vi "B_sweep_3ch_DR_v2.1.vi"(1 "name or relative path":string="Bsweeps_lockin_500mK_Vbg2.0V", 3 "description":string="SA02657K.20130302\ntemp=500mK\nVbg=1.9V\n25Oe/s scan rate", 5 "Stop":bool, 8 "slow scan through zero?":bool, 11 "sec to stablize B":u32=10, 15 "B Start (Oe)":dbl=-10000.0, 16 "B End (Oe)":dbl=10000.0, 17 "B Scan (Oe/sec)":dbl=25.0) -> (0 "Pickering":string="I-:5\nV2+:28\nI+:2\nV1+:3\nV-:4\nV2-:4\n", 10 "Zx 2":cluster{"Y":dbl[], "Y":dbl[]}(graph), 12 "Zx":cluster{"Y":dbl[], "Y":dbl[]}(graph), 13 "T":cluster{"Y":dbl[], "Y":dbl[]}(graph), 18 "Y Channel":cluster{"Y":dbl[], "Y":dbl[]}(graph), 19 "X Channel":cluster{"Y":dbl[], "Y":dbl[]}(graph))   [LabVIEW 2011]
uses:
  SubVI/ITX_Global.vi
  DAQ-lockin-SubVI/Source/Lock-in Globles.vi
panel:
  out "Current field (Oe)":dbl=9993.39
  in  "Tab Control":T1(tab)
  in  "Lock-in #":u16(ring) items=["Lock-in #1", "Lock-in #2", "Lock-in #3", "Lock-in #4"]
  in  "Lock-in # 3":u16(ring)=2 items=["Lock-in #1", "Lock-in #2", "Lock-in #3", "Lock-in #4"]
  in  "Lock-in # 4":u16(ring)=3 items=["Lock-in #1", "Lock-in #2", "Lock-in #3", "Lock-in #4"]
  in  "Device image":path=path "C:/Experiments/2011-summer Superconductivity-Spin Hall/Device images/SA02657K_20130302.png"
  out "Last Scan Image":T2(plugin-control)
  in  "Initial Rate (Oe/s)":i32=25
  in  "Stop Lockin":bool
  out "X 3":cluster{"Y":dbl[], "Y":dbl[]}(graph)
  out "Y 3":cluster{"Y":dbl[], "Y":dbl[]}(graph)
  out "X 4":cluster{"Y":dbl[], "Y":dbl[]}(graph)
  out "Y4":cluster{"Y":dbl[], "Y":dbl[]}(graph)
  out "Zy":cluster{"Y":dbl[], "Y":dbl[]}(graph)
  out "Zy 2":cluster{"Y":dbl[], "Y":dbl[]}(graph)
  # "yes"
  # "no"
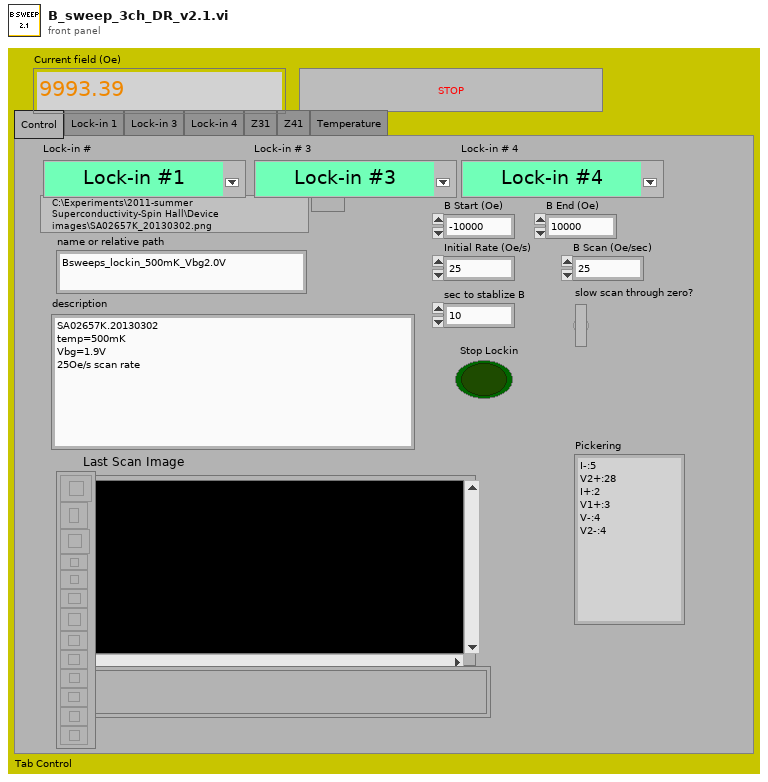
[diagram p1: front panel]
types:
  T1 = enum32{"Control", "Lock-in 1", "Lock-in 3", "Lock-in 4", "Z31", "Z41", "Temperature"}
  T2 = typedef "IMAQ Image.ctl" = refnum<image>
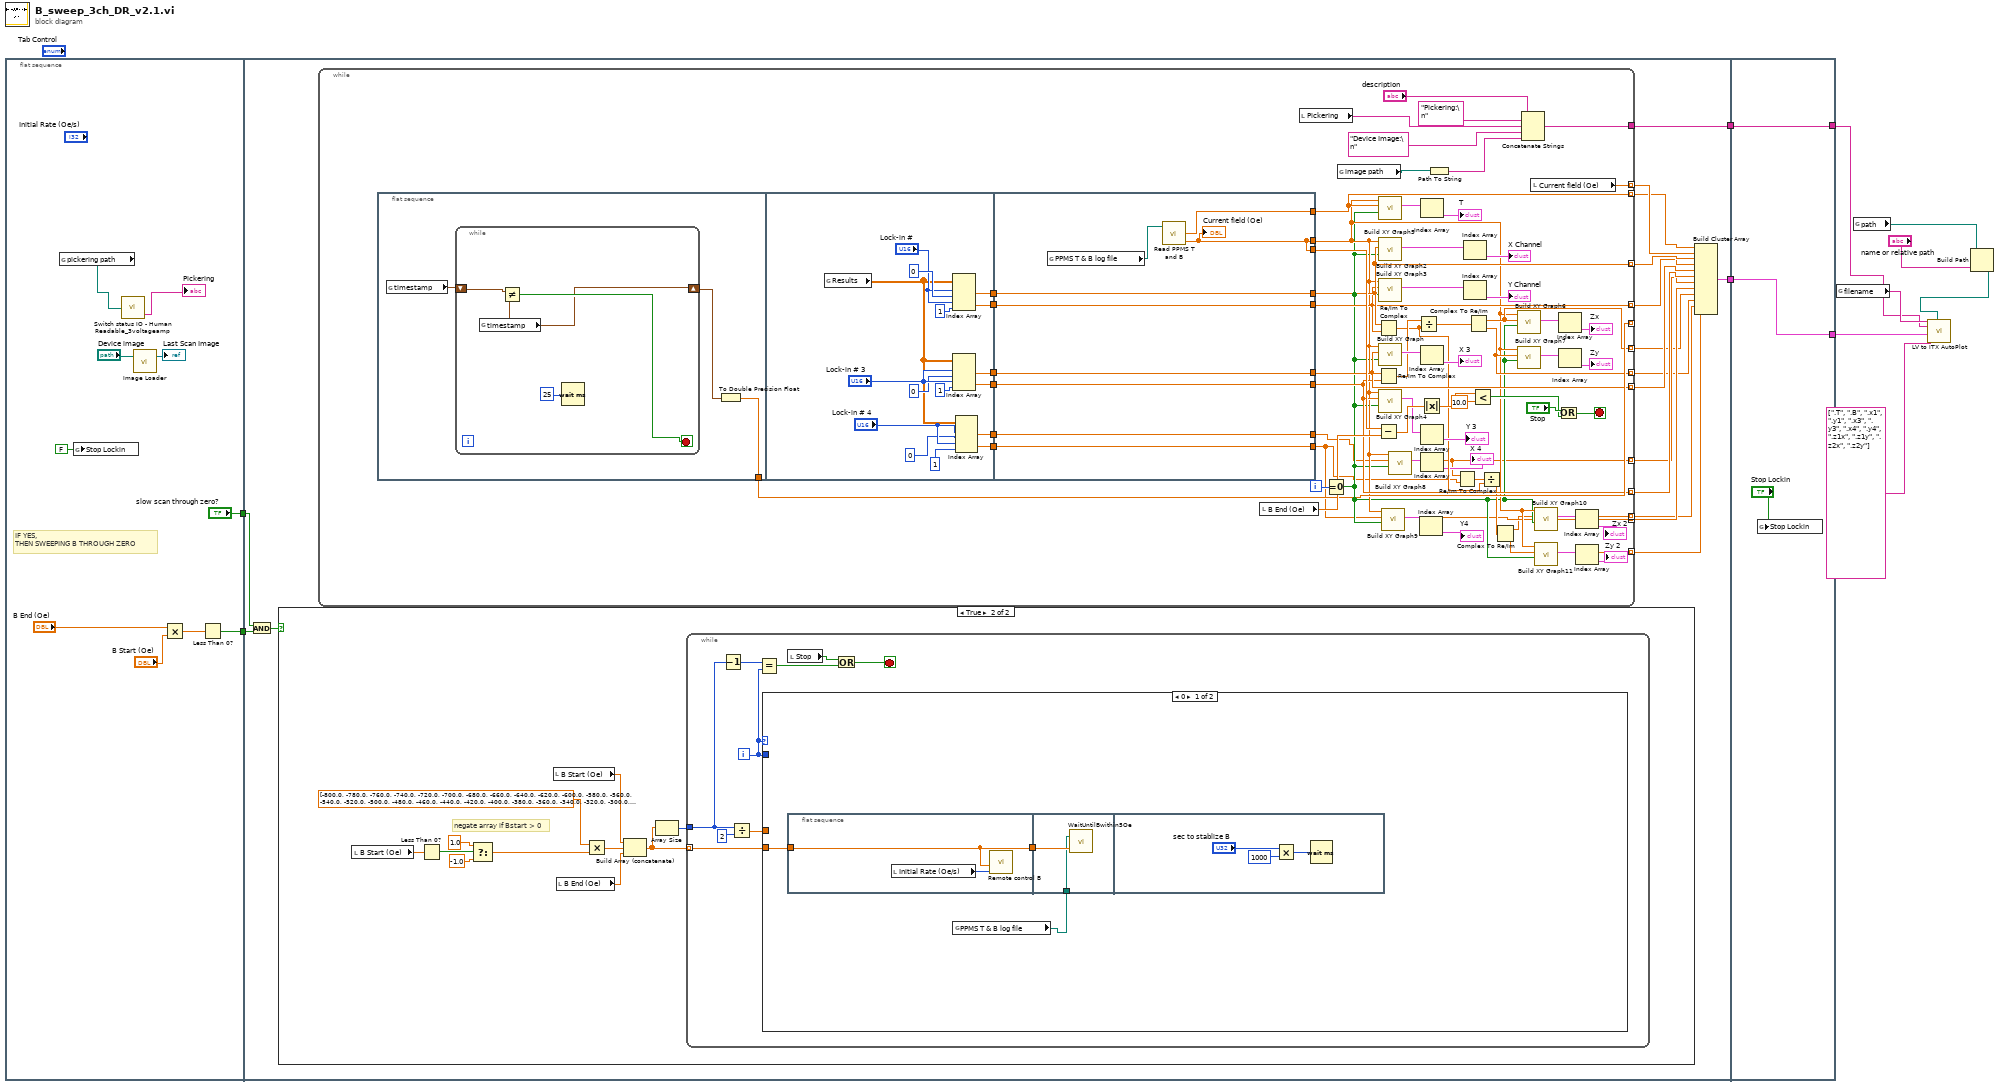
[diagram p0: block diagram]
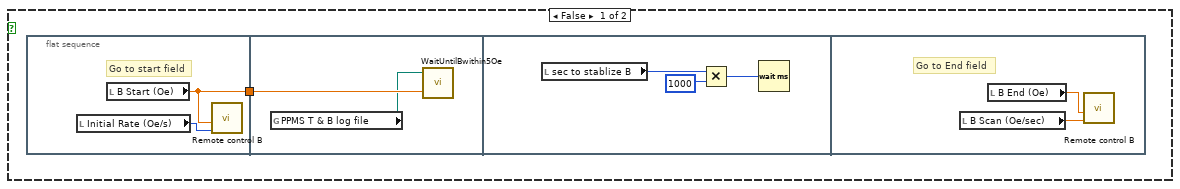
[diagram p2: hidden frame]
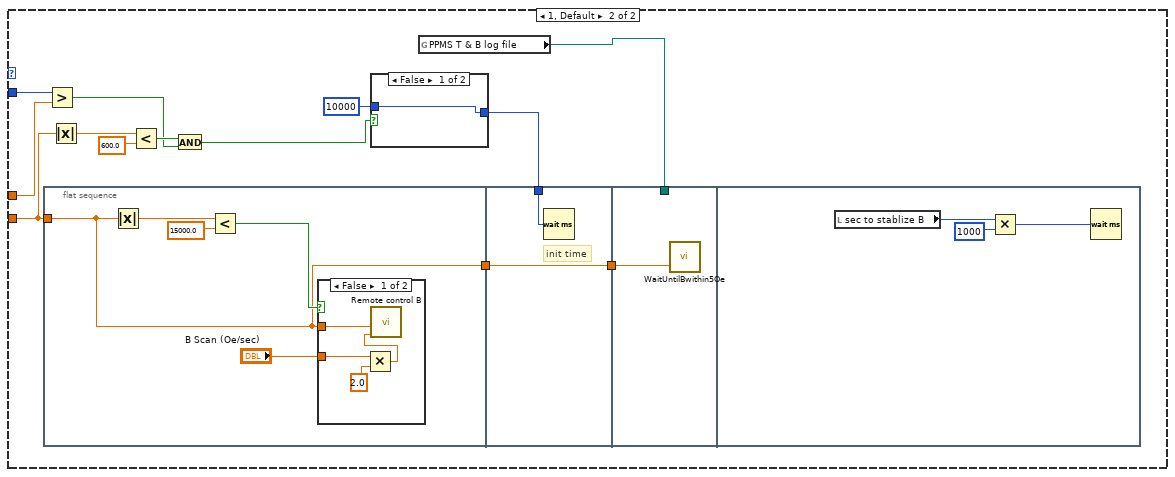
[diagram p3: hidden frame]
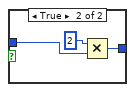
[diagram p4: hidden frame]
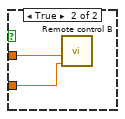
[diagram p5: hidden frame]
diagram:
  n1 = flat-sequence {
    tunnel: [w20] -> w11
    tunnel: ["slow scan through zero?"] -> w10
    tunnel: w11 -> [w38]
    tunnel: w10 -> [w37]
    tunnel: [w35] -> w7
    tunnel: [w22] -> w2
    tunnel: [w211] -> w4
    tunnel: w7 -> [w211]
    tunnel: [w209] -> w3
    tunnel: w2 -> [w209]
    frame #0 {
      # "IF YES,\nTHEN SWEEPING B THROUGH ZERO"
      n2 = global read "ITX_Global.vi" "pickering path"() -> (w13:path)
      n3 = global write "Lock-in Globles.vi" "Stop Lockin"(FALSE ("Stop Lockin")) -> ()
      n4 = call <userlib>:"Switch status IO - Human Readable_3voltageamp.vi"("Switch status"=w13) -> ("String"=→"Pickering":string)  [unwired: 3 in]
      n5 = call "Image Loader.vi"("File Path"="Device image") -> ("Last Scan Image"=→"Last Scan Image":T2)  [unwired: 2 in]
      n6 = Multiply(x="B End (Oe)", y="B Start (Oe)") -> (x*y=w21:dbl)
      n7 = Less Than 0?(x=w21) -> (x < 0?=w20:bool)
    }
    frame #1 {
      n8 = And(x=w37, y=w38) -> (x .and. y?=w36:bool)
      n9 = case shown="True" w36 {
        frame False {
          n10 = flat-sequence {
            tunnel: [w40] -> w39
            tunnel: w39 -> [w43]
            frame #0 {
              # "Go to start field"
              n11 = local read "Initial Rate (Oe/s)"() -> (w41:i32)
              n12 = local read "B Start (Oe)"() -> (w40:dbl)
              n13 = call "Remote control B.vi"("Rate (Oe/s)"=w41, "Field (Oe)"=w40) -> ()  [unwired: 7 in, 1 out]
            }
            frame #1 {
              n14 = global read "ITX_Global.vi" "PPMS T & B log file"() -> (w42:path)
              n15 = call "WaitUntilBwithin5Oe.vi"("Target Field (Oe)"=w43, "PPMS T & B log file"=w42) -> ()  [unwired: 2 in]
            }
            frame #2 {
              n16 = local read "sec to stablize B"() -> (w44:u32)
              n17 = Multiply(x=w44, y=u32 1000) -> (x*y=w45:u32)
              n18 = Wait (ms)(milliseconds to wait=w45) -> ()  [unwired: 1 out]
            }
            frame #3 {
              # "Go to End field"
              n19 = local read "B Scan (Oe/sec)"() -> (w47:dbl)
              n20 = local read "B End (Oe)"() -> (w48:dbl)
              n21 = call "Remote control B.vi"("Rate (Oe/s)"=w47, "Field (Oe)"=w48) -> ()  [unwired: 7 in, 1 out]
            }
          }
        }
        frame True {
          # "negate array if Bstart > 0"
          n22 = local read "B Start (Oe)"() -> (w59:dbl)
          n23 = Less Than 0?(x=w59) -> (x < 0?=w57:bool)
          n24 = Select(t=1.0, s=w57, f=-1.0) -> (s? t:f=w56:dbl)
          n25 = local read "B Start (Oe)"() -> (w51:dbl)
          n26 = local read "B End (Oe)"() -> (w52:dbl)
          n27 = Multiply(x=dbl[] [-800.0, -780.0, -760.0, -740.0, -720.0, -700.0, -680.0, -660.0, -640.0, -620.0, -600.0, -580.0, -560.0, -540.0, -520.0, -500.0, -480.0, -460.0, -440.0, -420.0, -400.0, -380.0, -360.0, -340.0, -320.0, -300.0, -280.0, -260.0, -240.0, -220.0, -200.0, -190.0, -180.0, -170.0, -160.0, -150.0, -140.0, -130.0, -120.0, -110.0, -100.0, -90.0, -80.0, -70.0, -60.0, -50.0, -40.0, -30.0, -20.0, -10.0, 0.0, 10.0, 20.0, 30.0, 40.0, 50.0, 60.0, 70.0, 80.0, 90.0, 100.0, 110.0, 120.0, 130.0, 140.0, 150.0, 160.0, 170.0, 180.0, 190.0, 200.0, 220.0, 240.0, 260.0, 280.0, 300.0, 320.0, 340.0, 360.0, 380.0, 400.0, 420.0, 440.0, 460.0, 480.0, 500.0, 520.0, 540.0, 560.0, 580.0, 600.0, 620.0, 640.0, 660.0, 680.0, 700.0, 720.0, 740.0, 760.0, 780.0, 800.0], y=w56) -> (x*y=w53:dbl[])
          n28 = Build Array (concatenate)(w51, w53, w52) -> (w50:dbl[])
          n29 = Array Size(array=w50) -> (size(s)=w49:i32)
          n30 = while {
            tunnel: w50 -> [w68] mode=indexing
            tunnel: w49 -> [w63]
            i -> [w60]
            stop <- w64 stop-if-true
            n31 = Decrement(x=w63) -> (x-1=w67:i32)
            n32 = Divide(x=w63, y=2) -> (x/y=w61:dbl)
            n33 = Equal?(x=w67, y=w60) -> (x = y?=w66:bool)
            n34 = case shown="0" w60 {
              tunnel: w68 -> [w70 w89]
              tunnel: w61 -> [_ w85]
              tunnel: w60 -> [_ w84]
              frame 0 {
                n35 = flat-sequence {
                  tunnel: w70 -> [w73]
                  tunnel: [w73] -> w71
                  tunnel: w69 -> [w74]
                  tunnel: w71 -> [w75]
                  frame #0 {
                    n36 = local read "Initial Rate (Oe/s)"() -> (w72:i32)
                    n37 = call "Remote control B.vi"("Rate (Oe/s)"=w72, "Field (Oe)"=w73) -> ()  [unwired: 7 in, 1 out]
                  }
                  frame #1 {
                    n38 = call "WaitUntilBwithin5Oe.vi"("Target Field (Oe)"=w75, "PPMS T & B log file"=w74) -> ()  [unwired: 2 in]
                  }
                  frame #2 {
                    n39 = Multiply(x="sec to stablize B", y=u32 1000) -> (x*y=w77:u32)
                    n40 = Wait (ms)(milliseconds to wait=w77) -> ()  [unwired: 1 out]
                  }
                }
                n41 = global read "ITX_Global.vi" "PPMS T & B log file"() -> (w69:path)
              }
              frame 1, Default {
                n42 = flat-sequence {
                  tunnel: w89 -> [w97]
                  tunnel: [w97] -> w91
                  tunnel: w91 -> [w108]
                  tunnel: [w108] -> w90
                  tunnel: w80 -> [w107]
                  tunnel: w79 -> [_]
                  tunnel: w90 -> [w109]
                  frame #0 {
                    n43 = Absolute Value(x=w97) -> (abs(x)=w96:dbl)
                    n44 = Less?(x=w96, y=15000.0) -> (x < y?=w98:bool)
                    n45 = case shown="False" w98 {
                      tunnel: w97 -> [w104 w106]
                      tunnel: "B Scan (Oe/sec)" -> [w103 w105]
                      frame False {
                        n46 = Multiply(x=w103, y=2.0) -> (x*y=w101:dbl)
                        n47 = call "Remote control B.vi"("Rate (Oe/s)"=w101, "Field (Oe)"=w104) -> ()  [unwired: 7 in, 1 out]
                      }
                      frame True {
                        n48 = call "Remote control B.vi"("Rate (Oe/s)"=w105, "Field (Oe)"=w106) -> ()  [unwired: 7 in, 1 out]
                      }
                    }
                  }
                  frame #1 {
                    # "init time"
                    n49 = Wait (ms)(milliseconds to wait=w107) -> ()  [unwired: 1 out]
                  }
                  frame #2 {
                    n50 = call "WaitUntilBwithin5Oe.vi"("Target Field (Oe)"=w109) -> ()  [unwired: 3 in]
                  }
                  frame #3 {
                    n51 = local read "sec to stablize B"() -> (w110:u32)
                    n52 = Multiply(x=w110, y=u32 1000) -> (x*y=w111:u32)
                    n53 = Wait (ms)(milliseconds to wait=w111) -> ()  [unwired: 1 out]
                  }
                }
                n54 = Greater?(x=w84, y=w85) -> (0:w83:bool)
                n55 = Absolute Value(x=w89) -> (abs(x)=w86:dbl)
                n56 = Less?(x=w86, y=600.0) -> (x < y?=w87:bool)
                n57 = And(x=w87, y=w83) -> (x .and. y?=w82:bool)
                n58 = case shown="False" w82 {
                  tunnel: u32 10000 ("y") -> [w92 w95]
                  tunnel: [w92 w93] -> w80
                  frame False {
                  }
                  frame True {
                    n59 = Multiply(x=u32 2, y=w95) -> (x*y=w93:u32)
                  }
                }
                n60 = global read "ITX_Global.vi" "PPMS T & B log file"() -> (w79:path)
              }
            }
            n61 = local read "Stop"() -> (w65:bool)
            n62 = Or(x=w65, y=w66) -> (x .or. y?=w64:bool)
          }
        }
      }
      n63 = while {
        tunnel: [w147] -> _ mode=indexing
        tunnel: [w146] -> w33 mode=indexing
        tunnel: [w145] -> w34 mode=indexing
        tunnel: [w144] -> w32 mode=indexing
        tunnel: [w143] -> w30 mode=indexing
        tunnel: [w142] -> w31 mode=indexing
        tunnel: [w141] -> w29 mode=indexing
        tunnel: [w140] -> w26 mode=indexing
        tunnel: [w139] -> w25 mode=indexing
        tunnel: [w117] -> w35
        tunnel: [w116] -> w28 mode=indexing
        tunnel: [w115] -> w27 mode=indexing
        tunnel: [w114] -> w24 mode=indexing
        tunnel: [w113] -> w23 mode=indexing
        i -> [w176]
        stop <- w169 stop-if-true
        n64 = flat-sequence {
          tunnel: [w179] -> w147
          tunnel: [w196] -> w151
          tunnel: [w195] -> w150
          tunnel: [w191] -> w149
          tunnel: [w190] -> w148
          tunnel: [w185] -> w138
          tunnel: [w184] -> w137
          tunnel: [w203] -> w127
          tunnel: [w203] -> w159
          tunnel: w151 -> [w208]
          tunnel: [w208] -> w142
          tunnel: w150 -> [w207]
          tunnel: [w207] -> w144
          tunnel: [w206] -> w143
          tunnel: w149 -> [w206]
          tunnel: w148 -> [w205]
          tunnel: [w205] -> w141
          tunnel: [w204] -> w146
          tunnel: [w202] -> w116
          tunnel: w138 -> [w202]
          tunnel: [w201] -> w115
          tunnel: w137 -> [w201]
          frame #0 {
            n65 = global read "Lock-in Globles.vi" "timestamp"() -> (w178:timestamp)
            n66 = while {
              shift-right: [w181] -> w177
              shift-left: w178 -> [w183]
              stop <- w182 stop-if-true
              n67 = global read "Lock-in Globles.vi" "timestamp"() -> (w181:timestamp)
              n68 = Not Equal?(x=w183, y=w181) -> (x != y?=w182:bool)
              n69 = Wait (ms)(milliseconds to wait=u32 25) -> ()  [unwired: 1 out]
            }
            n70 = To Double Precision Float(number=w177) -> (double precision float=w179:dbl)
          }
          frame #1 {
            n71 = global read "Lock-in Globles.vi" "Results"() -> (w186:dbl[][])
            n72 = Index Array(array=w186, index (row) #1="Lock-in #", index (col) #1=0 ("disabled index (col)"), index (row) #2="Lock-in #", index (col) #2=1 ("disabled index (col)")) -> (element #1=w195:dbl, element #2=w196:dbl)
            n73 = Index Array(array=w186, index (row) #1="Lock-in # 3", index (col) #1=0 ("disabled index (col)"), index (row) #2="Lock-in # 3", index (col) #2=1 ("disabled index (col)")) -> (element #1=w191:dbl, element #2=w190:dbl)
            n74 = Index Array(array=w186, index (row) #1="Lock-in # 4", index (col) #1=0 ("disabled index (col)"), index (row) #2="Lock-in # 4", index (col) #2=1 ("disabled index (col)")) -> (element #1=w185:dbl, element #2=w184:dbl)
          }
          frame #2 {
            n75 = global read "ITX_Global.vi" "PPMS T & B log file"() -> (w200:path)
            n76 = call "Read PPMS T and B.vi"("file (use dialog)"=w200) -> ("Field"=w203:dbl, "Temperature"=w204:dbl)  [unwired: 2 in, 1 out]
            "Current field (Oe)" <- w203
          }
        }
        n77 = local read "B End (Oe)"() -> (w160:dbl)
        n78 = local read "Pickering"() -> (w119:string)
        n79 = Equal To 0?(x=w176) -> (x = 0?=w126:bool)
        n80 = global read "ITX_Global.vi" "image path"() -> (w118:path)
        n81 = Re/Im To Complex(1:w142, 2:w144) -> (0:w135:cdb)
        n82 = Re/Im To Complex(1:w141, 2:w143) -> (0:w164:cdb)
        n83 = Subtract(x=w159, y=w160) -> (x-y=w174:dbl)
        n84 = call "Build XY Graph5"("Reset"=w126, "Y Input"=w146, "X Input"=w127) -> ("XY Graph"=w165:cluster{"Y":dbl[], "Y":dbl[]}[])  [unwired: 2 in, 6 out]
        n85 = call "Build XY Graph2"("Reset"=w126, "Y Input"=w144, "X Input"=w127) -> ("XY Graph"=w170:cluster{"Y":dbl[], "Y":dbl[]}[])  [unwired: 2 in, 6 out]
        n86 = call "Build XY Graph3"("Reset"=w126, "Y Input"=w142, "X Input"=w127) -> ("XY Graph"=w171:cluster{"Y":dbl[], "Y":dbl[]}[])  [unwired: 2 in, 6 out]
        n87 = call "Build XY Graph"("Reset"=w126, "Y Input"=w143, "X Input"=w127) -> ("XY Graph"=w167:cluster{"Y":dbl[], "Y":dbl[]}[])  [unwired: 2 in, 6 out]
        n88 = call "Build XY Graph4"("Reset"=w126, "Y Input"=w141, "X Input"=w127) -> ("XY Graph"=w166:cluster{"Y":dbl[], "Y":dbl[]}[])  [unwired: 2 in, 6 out]
        n89 = call "Build XY Graph9"("Reset"=w126, "Y Input"=w115, "X Input"=w127) -> ("XY Graph"=w131:cluster{"Y":dbl[], "Y":dbl[]}[])  [unwired: 2 in, 6 out]
        n90 = call "Build XY Graph8"("Reset"=w126, "Y Input"=w116, "X Input"=w127) -> ("XY Graph"=w133:cluster{"Y":dbl[], "Y":dbl[]}[])  [unwired: 2 in, 6 out]
        n91 = Divide(x=w164, y=w135) -> (x/y=w163:cdb)
        n92 = Index Array(array=w131) -> (element=→"Y4":cluster{"Y":dbl[], "Y":dbl[]})  [unwired: 1 in]
        n93 = Index Array(array=w165) -> (element=→"T":cluster{"Y":dbl[], "Y":dbl[]})  [unwired: 1 in]
        n94 = Index Array(array=w167) -> (element=→"X 3":cluster{"Y":dbl[], "Y":dbl[]})  [unwired: 1 in]
        n95 = Absolute Value(x=w174) -> (abs(x)=w173:dbl)
        n96 = Index Array(array=w166) -> (element=→"Y 3":cluster{"Y":dbl[], "Y":dbl[]})  [unwired: 1 in]
        n97 = Index Array(array=w133) -> (element=→"X 4":cluster{"Y":dbl[], "Y":dbl[]})  [unwired: 1 in]
        n98 = Path To String(path=w118) -> (string=w120:string)
        n99 = Re/Im To Complex(1:w115, 2:w116) -> (0:w136:cdb)
        n100 = Index Array(array=w170) -> (element=→"X Channel":cluster{"Y":dbl[], "Y":dbl[]})  [unwired: 1 in]
        n101 = Index Array(array=w171) -> (element=→"Y Channel":cluster{"Y":dbl[], "Y":dbl[]})  [unwired: 1 in]
        n102 = Complex To Re/Im(x + iy=w163) -> (x=w140:dbl, y=w139:dbl)
        n103 = Less?(x=w173, y=10.0) -> (x < y?=w168:bool)
        n104 = Divide(x=w136, y=w135) -> (x/y=w134:cdb)
        n105 = Complex To Re/Im(x + iy=w134) -> (x=w114:dbl, y=w113:dbl)
        n106 = call "Build XY Graph6"("Reset"=w126, "Y Input"=w140, "X Input"=w127) -> ("XY Graph"=w162:cluster{"Y":dbl[], "Y":dbl[]}[])  [unwired: 2 in, 6 out]
        n107 = call "Build XY Graph7"("Reset"=w126, "Y Input"=w139, "X Input"=w127) -> ("XY Graph"=w161:cluster{"Y":dbl[], "Y":dbl[]}[])  [unwired: 2 in, 6 out]
        n108 = Concatenate Strings("description", "Pickering:\n" ("string"), w119, "Device Image:\n" ("string"), w120) -> (w117:string)
        n109 = local read "Current field (Oe)"() -> (w145:dbl)
        n110 = call "Build XY Graph10"("Reset"=w126, "Y Input"=w114, "X Input"=w127) -> ("XY Graph"=w128:cluster{"Y":dbl[], "Y":dbl[]}[])  [unwired: 2 in, 6 out]
        n111 = call "Build XY Graph11"("Reset"=w126, "Y Input"=w113, "X Input"=w127) -> ("XY Graph"=w129:cluster{"Y":dbl[], "Y":dbl[]}[])  [unwired: 2 in, 6 out]
        n112 = Or(x="Stop", y=w168) -> (x .or. y?=w169:bool)
        n113 = Index Array(array=w162) -> (element=→"Zx":cluster{"Y":dbl[], "Y":dbl[]})  [unwired: 1 in]
        n114 = Index Array(array=w161) -> (element=→"Zy":cluster{"Y":dbl[], "Y":dbl[]})  [unwired: 1 in]
        n115 = Index Array(array=w128) -> (element=→"Zx 2":cluster{"Y":dbl[], "Y":dbl[]})  [unwired: 1 in]
        n116 = Index Array(array=w129) -> (element=→"Zy 2":cluster{"Y":dbl[], "Y":dbl[]})  [unwired: 1 in]
      }
      n117 = Build Cluster Array(w33, w34, w32, w31, w30, w29, w28, w27, w26, w25, w24, w23) -> (w22:cluster{dbl[]}[])
    }
    frame #2 {
      n118 = global write "Lock-in Globles.vi" "Stop Lockin"("Stop Lockin") -> ()
    }
  }
  n119 = global read "ITX_Global.vi" "filename"() -> (w5:string)
  n120 = global read "ITX_Global.vi" "path"() -> (w9:path)
  n121 = Build Path(base path=w9, name or relative path="name or relative path") -> (appended path=w6:path)
  n122 = call <userlib>:"LV to ITX AutoPlot.vi"("filename"=w5, "path"=w6, "Notes"=w4, "Data"=w3, "wavenames (.Vx, etc)"=string[] [".T", ".B", ".x1", ".y1", ".x3", ".y3", ".x4", ".y4", ".z1x", ".z1y", ".z2x", ".z2y"]) -> ()  [unwired: 10 in, 1 out]
